vi "timeinms.vi"() -> (3 "Date & Time With Milliseconds":string)   [LabVIEW 2010]
doc: "This VI displays the current date and time to the nearest millisecond by converting the output of the Get Date/Time In Seconds function into a string. The seconds output by this function include a fractional amount (milliseconds) that you can capture using the Quotient & Remainder function. You can then convert the number of milliseconds into a string and \"paste\" the milliseconds into the string that the Format Date/Time String function produces."
panel:
  # "Run the VI to capture the current date and time to the nearest millisecond in a string.\n\nSelect Help»Show Context Help and move the cursor over the VI icon to display help for this VI."
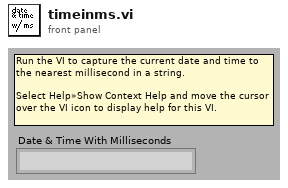
[diagram p1: front panel]
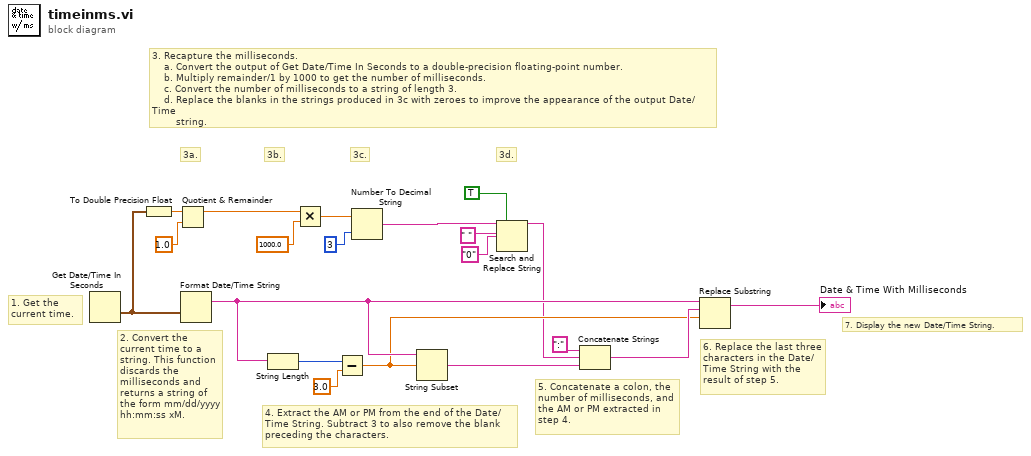
[diagram p0: block diagram]
diagram:
  # "3. Recapture the milliseconds.\n    a. Convert the output of Get Date/Time In Seconds to a double-precision floating-point number.\n    b. Multiply remainder/1 by 1000 to get the number of milliseconds.\n    c. Convert the number of milliseconds to a string of length 3.\n    d. Replace the blanks in the strings produced in 3c with zeroes to improve the appearance of the output Date/Time\n        string."
  # "7. Display the new Date/Time String."
  # "6. Replace the last three characters in the Date/Time String with the result of step 5."
  # "5. Concatenate a colon, the number of milliseconds, and the AM or PM extracted in step 4."
  # "3d."
  # "3c."
  # "3b."
  # "3a."
  # "4. Extract the AM or PM from the end of the Date/Time String. Subtract 3 to also remove the blank preceding the characters."
  # "2. Convert the current time to a string. This function discards the milliseconds and returns a string of the form mm/dd/yyyy hh:mm:ss xM."
  # "1. Get the current time."
  n1 = Get Date/Time In Seconds() -> (seconds since 1Jan1904=w6:timestamp)
  n2 = To Double Precision Float(number=w6) -> (double precision float=w9:dbl)
  n3 = Quotient & Remainder(x=w9, y=1.0) -> (x-y*floor(x/y)=w18:dbl)  [unwired: 1 out]
  n4 = Format Date/Time String(seconds (now)=w6) -> (date/time string=w12:string)  [unwired: 2 in]
  n5 = String Length(string=w12) -> (length=w20:i32)
  n6 = Multiply(x=w18, y=1000.0) -> (x*y=w8:dbl)
  n7 = Subtract(x=w20, y=3.0) -> (x-y=w10:dbl)
  n8 = Number To Decimal String(number=w8, width (-)=i16 3) -> (decimal integer string=w4:string)
  n9 = String Subset(string=w12, offset (0)=w10) -> (substring=w13:string)  [unwired: 1 in]
  n10 = Search and Replace String(replace all?=TRUE ("replace all? (F)"), input string=w4, search string=" ", replace string="0" ("replace string (\"\")")) -> (result string=w2:string)  [unwired: 4 in, 3 out]
  n11 = Concatenate Strings "Concatenate Strings"(":" ("string"), w2, w13) -> (w11:string)
  n12 = Replace Substring(3:w10, 4:w11, 5:w12) -> (1:→"Date & Time With Milliseconds":string)  [unwired: 1 in, 1 out]
